vi "Tilt alarm.vi"(0 "X-Array-Shift-in":dbl[](array[numeric]), 1 "Y-Array-Shift-in":dbl[](array[numeric]), 2 "X-Stored-Shift-in":dbl, 3 "Y-Stored-Shift-in":dbl, 4 "Grounded?":bool, 5 "Iterations":dbl, 6 "Filter?":bool, 7 "Accelerometer Ref X in":T1, 8 "Radius":dbl=5.0, 9 "Accelerometer Ref Y In":T1, 10 "high cutoff freq: fh":dbl=50.0) -> (14 "X-Array-Shift-out":dbl[](array[numeric]), 15 "Y-Array-Shift-out":dbl[](array[numeric]), 16 "X-Stored-Shift-out":dbl, 17 "Y-Stored-Shift-out":dbl, 18 "Alarm":bool)   [LabVIEW 2019]
uses:
  <vilib>/myRIO/Instrument Drivers/Onboard Devices/Accelerometer/typedefs/Accelerometer Reference.ctl
  <vilib>/myRIO/Common/Instrument Driver Framework/Utilities/typedefs/myRIO Generic Hardware Reference.ctl
  <vilib>/myRIO/Common/Instrument Driver Framework/Utilities/typedefs/Hardware Version Enum.ctl
  <vilib>/myRIO/Common/Instrument Driver Framework/Utilities/typedefs/myRIO v1.0 Reference.ctl
  <vilib>/myRIO/Common/Instrument Driver Framework/Utilities/typedefs/Generic FPGA Reference.ctl
  <vilib>/myRIO/Common/Instrument Driver Framework/myRIO v1.0/Accelerometer/typedefs/Accelerometer Channels List.ctl
  <vilib>/myRIO/Common/Instrument Driver Framework/myRIO v1.0/Accelerometer/typedefs/Accelerometer Channels Enum.ctl
  <vilib>/Analysis/3filter.llb/Filter Passband Type.ctl
  <vilib>/Utility/error.llb/Error Cluster From Error Code.vi
  <vilib>/myRIO/Common/Instrument Driver Framework/myRIO v1.0/Accelerometer/vis/myRIO v1.0 Read Accelerometer.vi
  <vilib>/Analysis/3filter.llb/Butterworth Filter (DBL).vi
  <vilib>/myRIO/Instrument Drivers/Onboard Devices/Accelerometer/Accelerometer.lvlib
  <vilib>/Analysis/NI_AALBase.lvlib
panel:
  out "X-Actual":dbl
  out "Y-Actual":dbl
  out "Y-Stored":dbl
  out "X-Stored":dbl
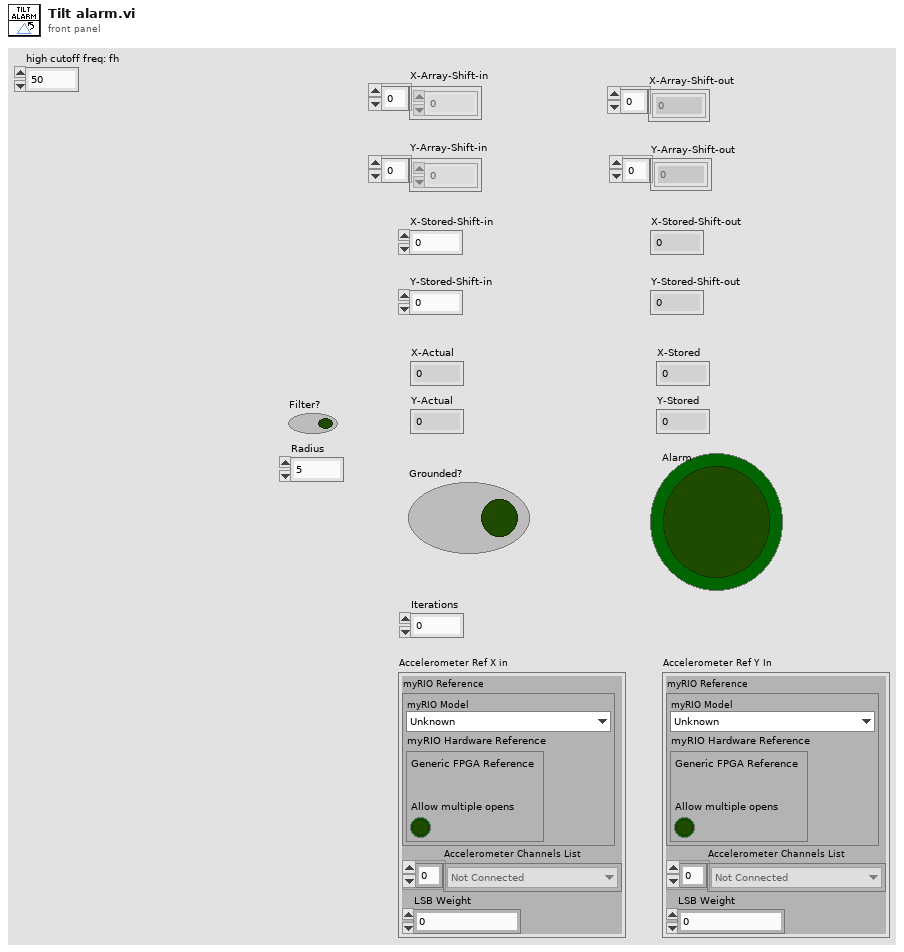
[diagram p1: front panel]
types:
  T1 = typedef "Accelerometer.lvlib/Accelerometer Reference.ctl" = cluster{"myRIO Reference":T2, "Accelerometer Channels List":T6, "LSB Weight":dbl}
  T2 = typedef "myRIO Generic Hardware Reference.ctl" = cluster{"myRIO Model":T3, "myRIO Hardware Reference":T4}
  T3 = typedef "Hardware Version Enum.ctl" = enum16{"Unknown", "myRIO-1900", "myRIO-1950", "roboRIO", "NI ELVIS RIO CM", "ELVIS III"}
  T4 = typedef "myRIO v1.0 Reference.ctl" = cluster{"Generic FPGA Reference":T5, "Allow multiple opens":bool}
  T5 = typedef "Generic FPGA Reference.ctl" = refnum<k20>
  T6 = typedef "Accelerometer Channels List.ctl" = T7[]
  T7 = typedef "Accelerometer Channels Enum.ctl" = enum16{"Not Connected", "X-Axis", "Y-Axis", "Z-Axis"}
  T8 = typedef "NI_AALBase.lvlib/Filter Passband Type.ctl" = enum32{"Lowpass", "Highpass", "Bandpass", "Bandstop"}
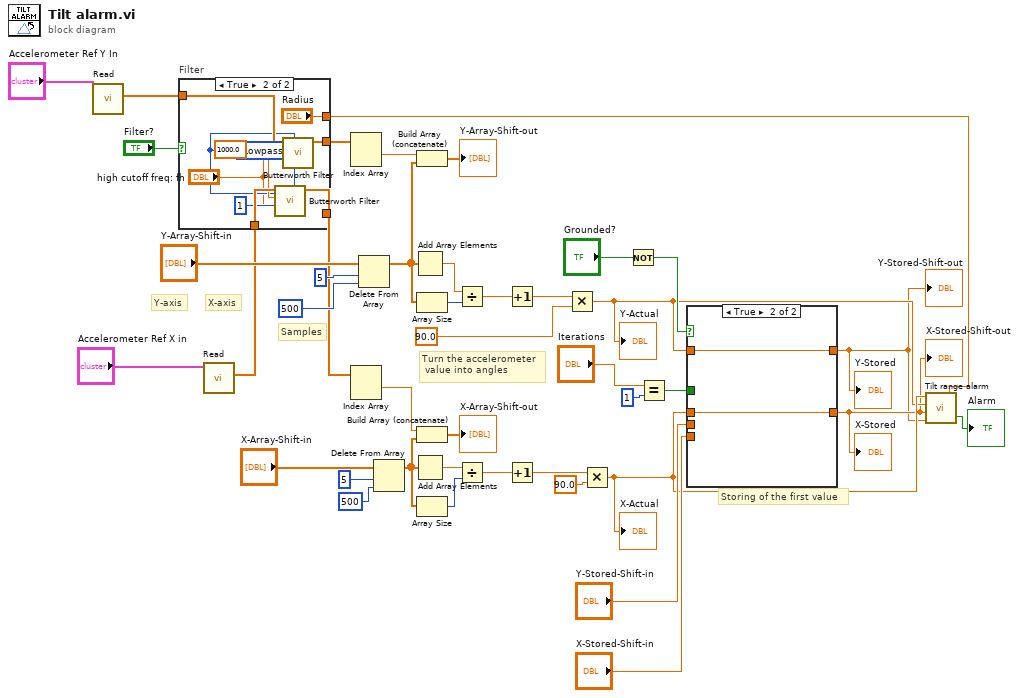
[diagram p0: block diagram]
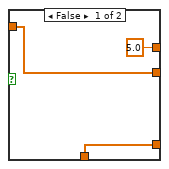
[diagram p2: hidden frame]
diagram:
  # "Storing of the first value"
  # "Turn the accelerometer\n value into angles"
  # "Samples"
  # "Y-axis"
  # "X-axis"
  n1 = call <vilib>:"Read.vi"("Accelerometer Ref In"="Accelerometer Ref Y In") -> ("Values"=w4:dbl[])  [unwired: 8 in, 2 out]
  n2 = call <vilib>:"Read.vi"("Accelerometer Ref In"="Accelerometer Ref X in") -> ("Values"=w6:dbl[])  [unwired: 8 in, 2 out]
  n3 = case "Filter" shown="True" "Filter?" {
    tunnel: w6 -> [w45 w54]
    tunnel: [w45 w53] -> w5
    tunnel: w4 -> [w44 w52]
    tunnel: [w44 w51] -> w3
    tunnel: [5.0 ("Radius") "Radius"] -> w1
    frame False {
    }
    frame True {
      w48 = 1 ("order")
      w49 = Filter_Passband_Type."Lowpass" ("filter type")
      w50 = 1000.0 ("sampling freq: fs")
      n4 = call-poly <vilib>:"Butterworth Filter.vi"("order"=w48, "filter type"=w49, "high cutoff freq: fh"="high cutoff freq: fh", "sampling freq: fs"=w50, "X"=w54) -> ("Filtered X"=w53:dbl[])  [unwired: 3 in, 1 out]
      n5 = call-poly <vilib>:"Butterworth Filter.vi"("order"=w48, "filter type"=w49, "high cutoff freq: fh"="high cutoff freq: fh", "sampling freq: fs"=w50, "X"=w52) -> ("Filtered X"=w51:dbl[])  [unwired: 3 in, 1 out]
    }
  }
  n6 = Index Array(array=w3) -> (element #1=w12:dbl)  [unwired: 2 in, 1 out]
  n7 = Index Array(array=w5) -> (element #1=w42:dbl)  [unwired: 2 in, 1 out]
  n8 = Delete From Array(array="Y-Array-Shift-in", length=5, index=500) -> (array with subset deleted=w35:dbl[])  [unwired: 1 out]
  n9 = Delete From Array(array="X-Array-Shift-in", length=5, index=500) -> (array with subset deleted=w33:dbl[])  [unwired: 1 out]
  n10 = Add Array Elements(numeric array=w35) -> (sum=w37:dbl)
  n11 = Add Array Elements(numeric array=w33) -> (sum=w34:dbl)
  n12 = Build Array (concatenate)(w12, w35) -> (→"Y-Array-Shift-out":dbl[])
  n13 = Array Size(array=w35) -> (size(s)=w36:i32)
  n14 = Build Array (concatenate)(w42, w33) -> (→"X-Array-Shift-out":dbl[])
  n15 = Array Size(array=w33) -> (size(s)=w32:i32)
  n16 = Divide(x=w37, y=w36) -> (x/y=w28:dbl)
  n17 = Divide(x=w34, y=w32) -> (x/y=w27:dbl)
  n18 = Increment(x=w28) -> (x+1=w29:dbl)
  n19 = Increment(x=w27) -> (x+1=w26:dbl)
  n20 = Multiply(x=w29, y=90.0) -> (x*y=w10:dbl)
  "Y-Actual" <- w10
  n21 = Multiply(x=w26, y=90.0) -> (x*y=w11:dbl)
  "X-Actual" <- w11
  n22 = Not(x="Grounded?") -> (.not. x?=w14:bool)
  n23 = Equal?(x="Iterations", y=1) -> (x = y?=w24:bool)
  n24 = case shown="True" w14 {
    tunnel: w11 -> [w56 w67]
    tunnel: w10 -> [w55 w66]
    tunnel: [w57 w67] -> w9
    tunnel: [w59 w66] -> w8
    tunnel: "X-Stored-Shift-in" -> [w58 _]
    tunnel: "Y-Stored-Shift-in" -> [w60 _]
    tunnel: w24 -> [w61 _]
    frame False {
      n25 = case shown="True" w61 {
        tunnel: w60 -> [w63 _]
        tunnel: [w63 w64] -> w59
        tunnel: w58 -> [w62 _]
        tunnel: [w62 w65] -> w57
        tunnel: w56 -> [_ w65]
        tunnel: w55 -> [_ w64]
        frame False {
        }
        frame True {
        }
      }
    }
    frame True {
    }
  }
  "X-Stored-Shift-out" <- w9
  "Y-Stored-Shift-out" <- w8
  "X-Stored" <- w9
  "Y-Stored" <- w8
  n26 = call "Tilt range alarm.vi"("Radius"=w1, "Y-Stored"=w8, "X-Stored"=w9, "Y-Actual"=w10, "X-Actual"=w11) -> ("Alarm"=→"Alarm":bool)
